vi "Stop.vi"(8 "error in (no error)":errorcluster) -> (0 "error out":errorcluster)   [LabVIEW 2015, in "G 5.lvlib"]
uses:
  G 5.lvlib
  AMTIUSBDevice.dll
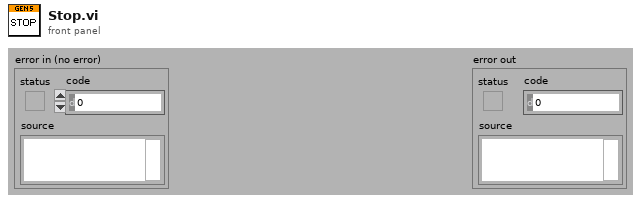
[diagram p1: front panel]
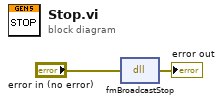
[diagram p0: block diagram]
diagram:
  n1 = dll-call lib="AMTIUSBDevice.dll" fn="fmBroadcastStop" label="Stop"(error in="error in (no error)") -> (error out=→"error out":errorcluster)  [unwired: 3 in, 1 out]
